vi "DataTable to arrayStr.vi"(5 "Online_Table":T1) -> (2 "appended array":string[](array[string]))   [LabVIEW 2014]
uses:
  Type'def/Online_Table.ctl
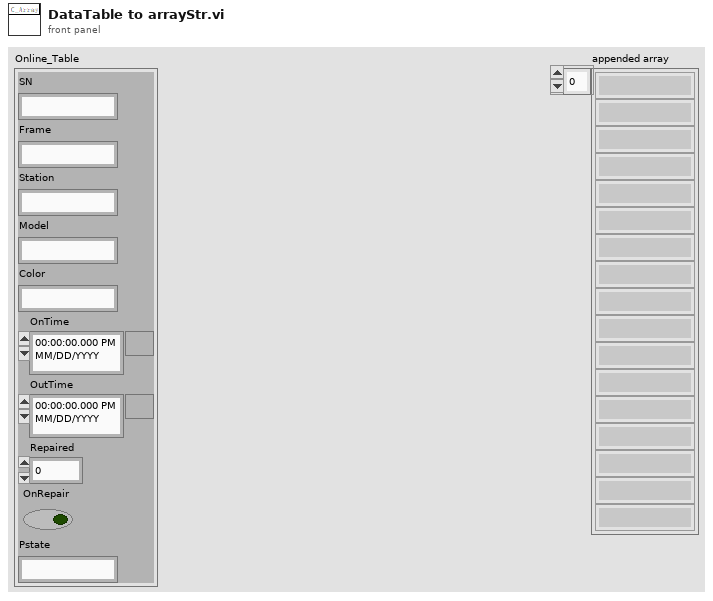
[diagram p1: front panel]
types:
  T1 = typedef "Online_Table.ctl" = cluster{"SN":string, "Frame":string, "Station":string, "Model":string, "Color":string, "OnTime":timestamp, "OutTime":timestamp, "Repaired":i32, "OnRepair":bool, "Pstate":string}
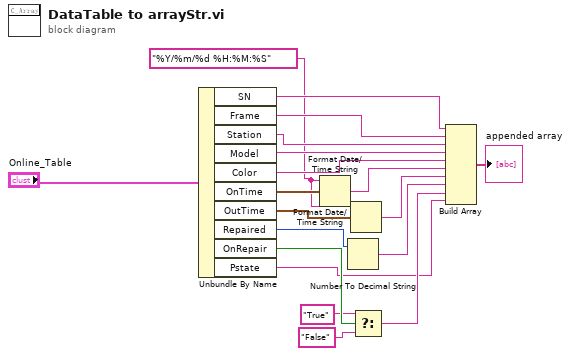
[diagram p0: block diagram]
diagram:
  w1 = "%Y/%m/%d %H:%M:%S"
  n1 = Unbundle By Name("Online_Table") -> ("SN"=w18:string, "Frame"=w17:string, "Station"=w16:string, "Model"=w15:string, "Color"=w14:string, "OnTime"=w13:timestamp, "OutTime"=w11:timestamp, "Repaired"=w9:i32, "OnRepair"=w7:bool, "Pstate"=w3:string)
  n2 = Format Date/Time String(time format string (%c)=w1, seconds (now)=w13) -> (date/time string=w12:string)  [unwired: 1 in]
  n3 = Number To Decimal String(number=w9) -> (decimal integer string=w8:string)  [unwired: 1 in]
  n4 = Format Date/Time String(time format string (%c)=w1, seconds (now)=w11) -> (date/time string=w10:string)  [unwired: 1 in]
  n5 = Select(t="True", s=w7, f="False") -> (s? t:f=w4:string)
  n6 = Build Array(w18, w17, w16, w15, w14, w12, w10, w8, w4, w3) -> (→"appended array":string[])
